vi "Fix Angle Align.vi"(11 "Right Setpoint":dbl) -> (3 "Fixed Angle":dbl)   [LabVIEW 2016]
uses:
  NavX/NavX Global.vi
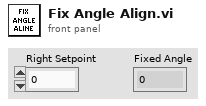
[diagram p1: front panel]
types:
  T1 = cluster{"Yaw":dbl, "Roll":dbl, "Pitch":dbl, "Heading":dbl, "Fused Heading":dbl}
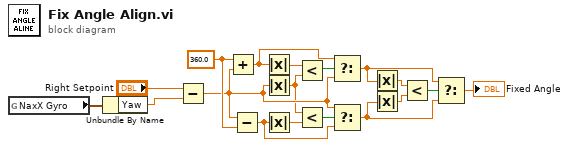
[diagram p0: block diagram]
diagram:
  w15 = 360.0 ("x")
  n1 = global read "NavX Global.vi" "NaxX Gyro"() -> (w16:T1)
  n2 = Unbundle By Name(w16) -> ("Yaw"=w18:dbl)
  n3 = Subtract(x="Right Setpoint", y=w18) -> (x-y=w9:dbl)
  n4 = Add(x=w15, y=w9) -> (x+y=w12:dbl)
  n5 = Subtract(x=w9, y=w15) -> (x-y=w7:dbl)
  n6 = Absolute Value(x=w12) -> (abs(x)=w14:dbl)
  n7 = Absolute Value(x=w9) -> (abs(x)=w8:dbl)
  n8 = Absolute Value(x=w7) -> (abs(x)=w10:dbl)
  n9 = Less?(x=w14, y=w8) -> (x < y?=w13:bool)
  n10 = Less?(x=w8, y=w10) -> (x < y?=w11:bool)
  n11 = Select(t=w12, s=w13, f=w9) -> (s? t:f=w4:dbl)
  n12 = Select(t=w9, s=w11, f=w7) -> (s? t:f=w2:dbl)
  n13 = Absolute Value(x=w4) -> (abs(x)=w5:dbl)
  n14 = Absolute Value(x=w2) -> (abs(x)=w6:dbl)
  n15 = Less?(x=w5, y=w6) -> (x < y?=w3:bool)
  n16 = Select(t=w4, s=w3, f=w2) -> (s? t:f=→"Fixed Angle":dbl)
